vi "reset.vi"(8 "error in (no error)":errorcluster, 11 "GenericImageAssembler in":refnum<class "GenericImageAssembler.lvclass">) -> (0 "error out":errorcluster, 3 "GenericImageAssembler out":refnum<class "GenericImageAssembler.lvclass">)   [LabVIEW 2010]
uses:
  class_data.vi
  GenericImageAssembler.lvclass
  common/classes/Image/Image/Image.lvclass
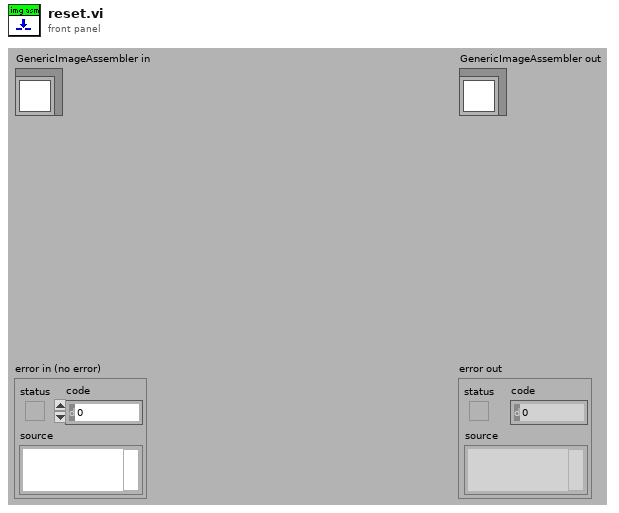
[diagram p1: front panel]
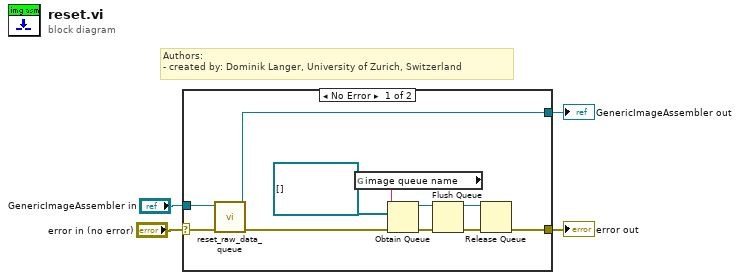
[diagram p0: block diagram]
diagram:
  # "Authors: \n- created by: Dominik Langer, University of Zurich, Switzerland"
  n1 = case shown="No Error" "error in (no error)" {
    selector: "error in (no error)" -> [w8 w17]
    tunnel: [w12 w17] -> w3
    tunnel: [w5 w16] -> w1
    tunnel: "GenericImageAssembler in" -> [w6 w16]
    frame No Error {
      n2 = call-dynamic "reset_raw_data_queue.vi"("error in (no error)"=w8, "GenericToplevelComponent in"=w6) -> ("error out"=w7:errorcluster, "GenericToplevelComponent out"=w5:refnum<class "GenericImageAssembler.lvclass">)  [unwired: 8 in]
      n3 = global read "class_data.vi" "image queue name"() -> (w15:string)
      n4 = Obtain Queue(name (unnamed)=w15, element data type=refnum<class "Image.lvclass">[] [], error in (no error)=w7) -> (queue out=w11:refnum<queue>, error out=w14:errorcluster)  [unwired: 2 in, 1 out]
      n5 = Flush Queue(queue=w11, error in (no error)=w14) -> (queue out=w10:refnum<queue>, error out=w13:errorcluster)  [unwired: 1 out]
      n6 = Release Queue(queue=w10, error in (no error)=w13) -> (error out=w12:errorcluster)  [unwired: 1 in, 2 out]
    }
    frame Error {
    }
  }
  "error out" <- w3
  "GenericImageAssembler out" <- w1
